vi "MeasLeakRate02.vi"() -> ()   [LabVIEW 2011]
panel:
  out "leak rate (Torr/min)":string
  out "S20":dbl
  out "S11":dbl
  out "S10":dbl
  out "S01":dbl
  out "S00":dbl
  out "A11":dbl[](array[numeric])
  out "P":dbl
  in  "first":bool=TRUE
  out "A20":dbl[](array[numeric])
  out "A10":dbl[](array[numeric])
  out "A01":dbl[](array[numeric])
  out "A00":dbl[](array[numeric])
  in  "interval (s)":dbl=0.5
  in  "stop":bool
  out "P(Torr)":string
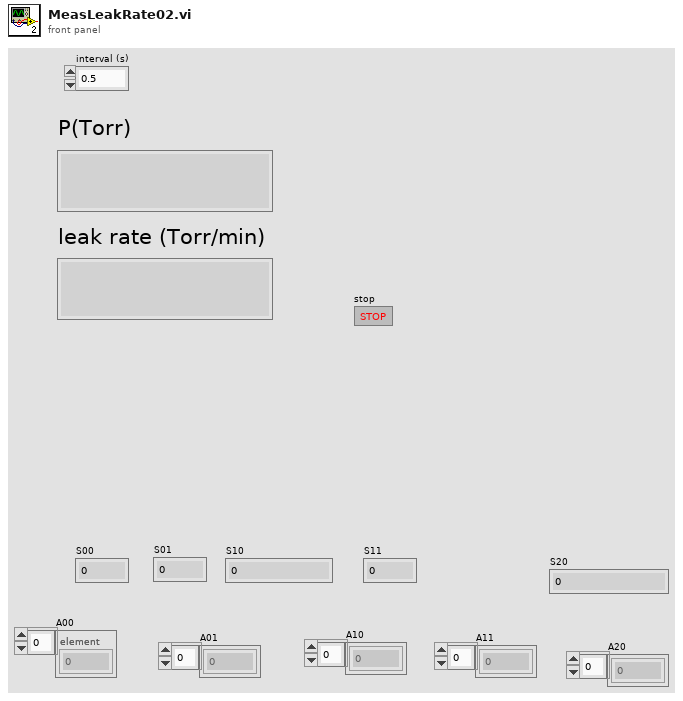
[diagram p1: front panel]
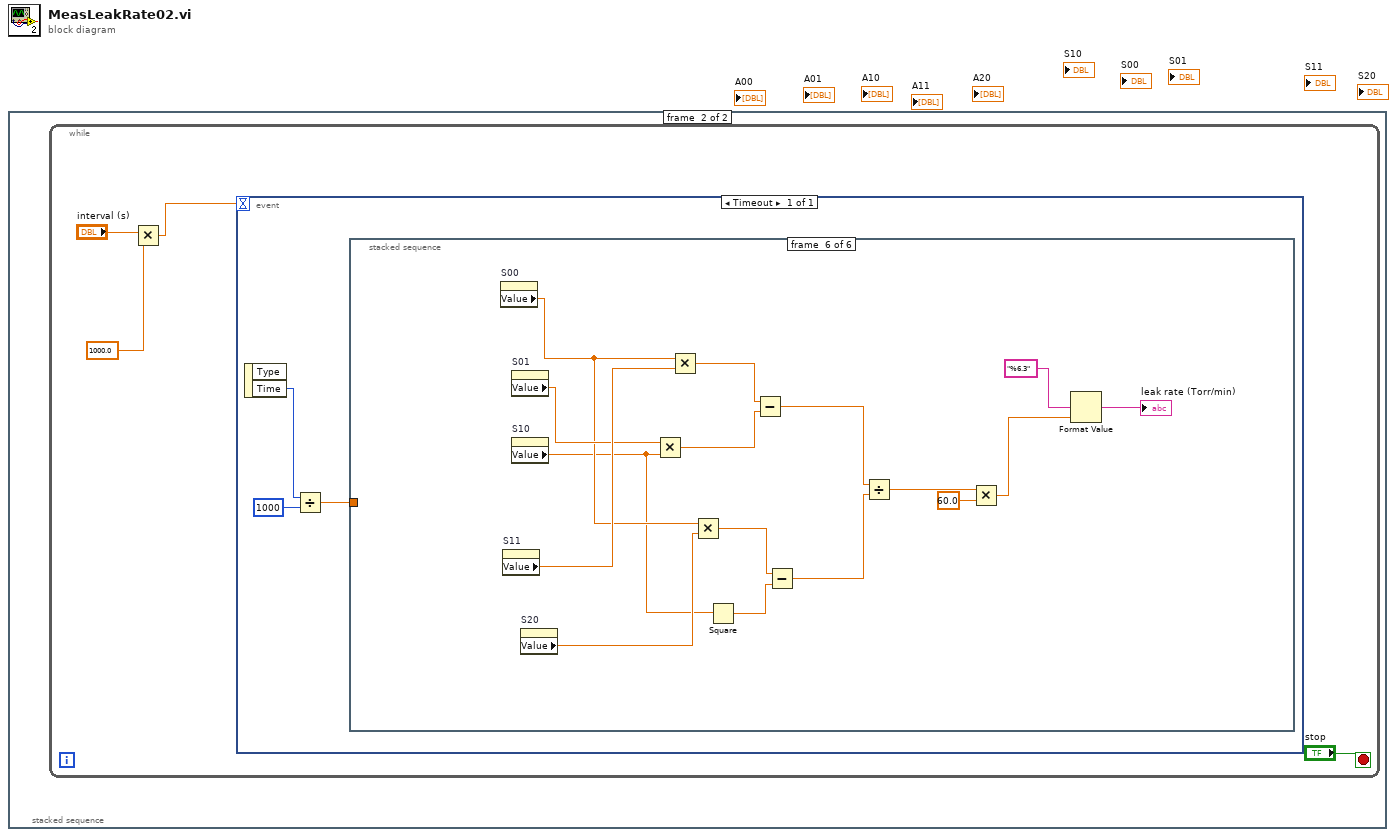
[diagram p0: block diagram]
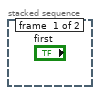
[diagram p2: hidden frame]
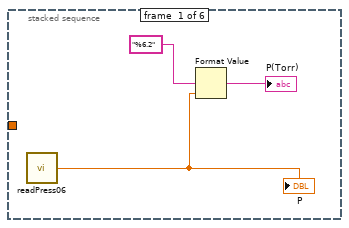
[diagram p3: hidden frame]
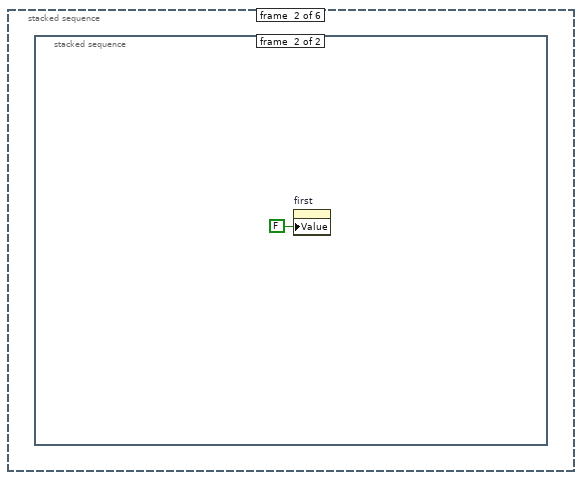
[diagram p4: hidden frame]
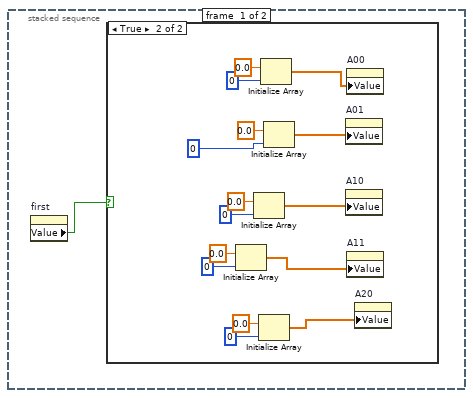
[diagram p5: hidden frame]
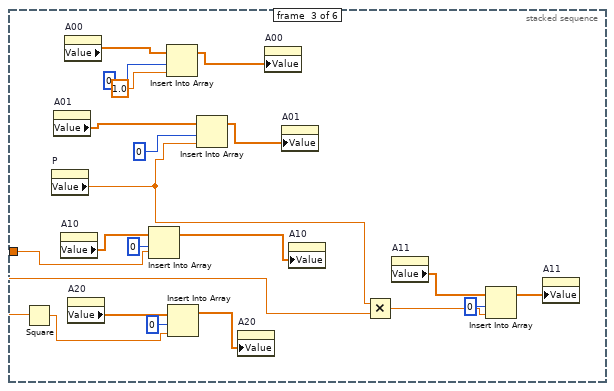
[diagram p7: hidden frame]
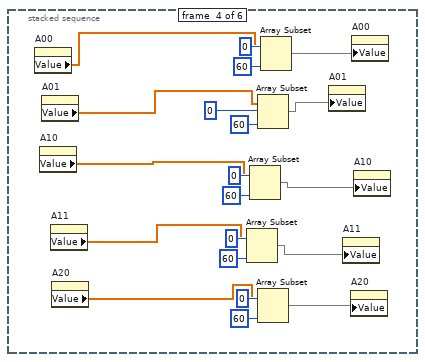
[diagram p8: hidden frame]
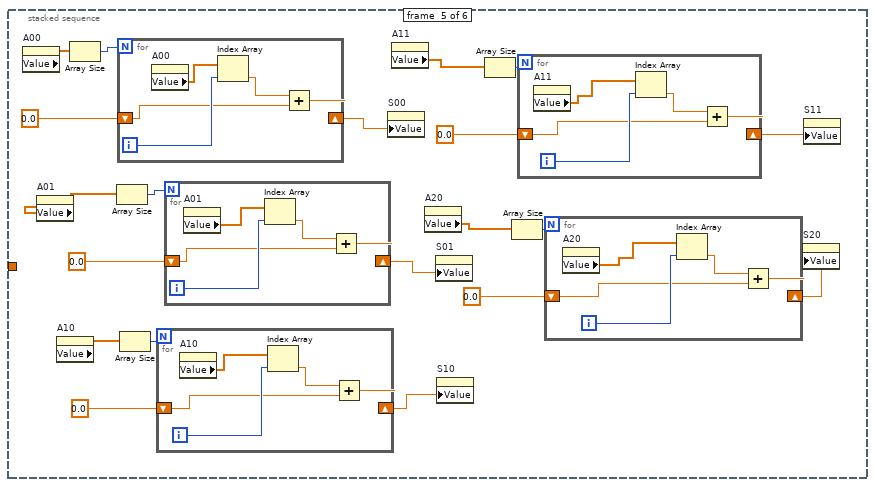
[diagram p9: hidden frame]
diagram:
  n1 = stacked-sequence {
    frame #0 {
    }
    frame #1 {
      n2 = while {
        stop <- "stop" stop-if-true
        n3 = Multiply(x="interval (s)", y=1000.0) -> (x*y=w2:dbl)
        n4 = event shown="[0] Timeout" {
          selector: _ -> [_]
          dyn-events: _ -> [_]
          timeout: w2 -> [_]
          event Timeout {
            n5 = event-data() -> ("Time"=w7:u32)  [unwired: 1 in, 1 out]
            n6 = Divide(x=w7, y=u32 1000) -> (x/y=w5:dbl)
            n7 = stacked-sequence {
              tunnel: w5 -> [_ _ w37 _ _ _]
              frame #0 {
                n8 = call "readPress06.vi"() -> ("P"=w9:dbl)
                "P" <- w9
                n9 = Format Value(format string="%6.2", value (0)=w9) -> (output string=→"P(Torr)":string)  [unwired: 1 in]
              }
              frame #1 {
                n10 = stacked-sequence {
                  frame #0 {
                    n11 = property on="first" class="Bool (strict)"() -> ("Value"=w11:bool)  [unwired: 2 in, 2 out]
                    n12 = case shown="True" w11 {
                      frame False {
                      }
                      frame True {
                        n13 = Initialize Array(0.0 ("element"), 0 ("dimension size")) -> (w14:dbl[])
                        n14 = Initialize Array(0.0 ("element"), 0 ("dimension size")) -> (w15:dbl[])
                        n15 = Initialize Array(0.0 ("element"), 0 ("dimension size")) -> (w13:dbl[])
                        n16 = Initialize Array(0.0 ("element"), 0 ("dimension size")) -> (w12:dbl[])
                        n17 = Initialize Array(0.0 ("element"), 0 ("dimension size")) -> (w16:dbl[])
                        n18 = property on="A01" class="Arr (strict)"("Value"=w16) -> ()  [unwired: 2 in, 2 out]
                        n19 = property on="A10" class="Arr (strict)"("Value"=w15) -> ()  [unwired: 2 in, 2 out]
                        n20 = property on="A00" class="Arr (strict)"("Value"=w12) -> ()  [unwired: 2 in, 2 out]
                        n21 = property on="A11" class="Arr (strict)"("Value"=w14) -> ()  [unwired: 2 in, 2 out]
                        n22 = property on="A20" class="Arr (strict)"("Value"=w13) -> ()  [unwired: 2 in, 2 out]
                      }
                    }
                  }
                  frame #1 {
                    n23 = property on="first" class="Bool (strict)"("Value"=FALSE ("first")) -> ()  [unwired: 2 in, 2 out]
                  }
                }
              }
              frame #2 {
                n24 = Square(x=w37) -> (x^2=w38:dbl)
                n25 = property on="P" class="DigNum (strict)"() -> ("Value"=w36:dbl)  [unwired: 2 in, 2 out]
                n26 = property on="A01" class="Arr (strict)"() -> ("Value"=w43:dbl[])  [unwired: 2 in, 2 out]
                n27 = property on="A10" class="Arr (strict)"() -> ("Value"=w42:dbl[])  [unwired: 2 in, 2 out]
                n28 = property on="A00" class="Arr (strict)"() -> ("Value"=w45:dbl[])  [unwired: 2 in, 2 out]
                n29 = property on="A20" class="Arr (strict)"() -> ("Value"=w40:dbl[])  [unwired: 2 in, 2 out]
                n30 = Insert Into Array(array=w42, index=0, new element=w37) -> (w30:dbl[])
                n31 = Insert Into Array(array=w45, index=0, new element=1.0 ("new element/subarray")) -> (w32:dbl[])
                n32 = Insert Into Array(array=w40, index=0, new element=w38) -> (w31:dbl[])
                n33 = Insert Into Array(array=w43, index=0, new element=w36) -> (w28:dbl[])
                n34 = property on="A20" class="Arr (strict)"("Value"=w31) -> ()  [unwired: 2 in, 2 out]
                n35 = property on="A00" class="Arr (strict)"("Value"=w32) -> ()  [unwired: 2 in, 2 out]
                n36 = property on="A01" class="Arr (strict)"("Value"=w28) -> ()  [unwired: 2 in, 2 out]
                n37 = property on="A10" class="Arr (strict)"("Value"=w30) -> ()  [unwired: 2 in, 2 out]
                n38 = Multiply(x=w36, y=w37) -> (x*y=w34:dbl)
                n39 = property on="A11" class="Arr (strict)"() -> ("Value"=w35:dbl[])  [unwired: 2 in, 2 out]
                n40 = Insert Into Array(array=w35, index=0, new element=w34) -> (w29:dbl[])
                n41 = property on="A11" class="Arr (strict)"("Value"=w29) -> ()  [unwired: 2 in, 2 out]
              }
              frame #3 {
                n42 = property on="A00" class="Arr (strict)"() -> ("Value"=w62:dbl[])  [unwired: 2 in, 2 out]
                n43 = property on="A10" class="Arr (strict)"() -> ("Value"=w53:dbl[])  [unwired: 2 in, 2 out]
                n44 = property on="A01" class="Arr (strict)"() -> ("Value"=w54:dbl[])  [unwired: 2 in, 2 out]
                n45 = property on="A11" class="Arr (strict)"() -> ("Value"=w52:dbl[])  [unwired: 2 in, 2 out]
                n46 = property on="A20" class="Arr (strict)"() -> ("Value"=w65:dbl[])  [unwired: 2 in, 2 out]
                n47 = Array Subset(array=w52, index=0, length=60) -> (w49:dbl[])
                n48 = Array Subset(array=w53, index=0, length=60) -> (w50:dbl[])
                n49 = Array Subset(array=w54, index=0, length=60) -> (w51:dbl[])
                n50 = Array Subset(array=w65, index=0, length=60) -> (w48:dbl[])
                n51 = Array Subset(array=w62, index=0, length=60) -> (w61:dbl[])
                n52 = property on="A01" class="Arr (strict)"("Value"=w51) -> ()  [unwired: 2 in, 2 out]
                n53 = property on="A11" class="Arr (strict)"("Value"=w49) -> ()  [unwired: 2 in, 2 out]
                n54 = property on="A20" class="Arr (strict)"("Value"=w48) -> ()  [unwired: 2 in, 2 out]
                n55 = property on="A00" class="Arr (strict)"("Value"=w61) -> ()  [unwired: 2 in, 2 out]
                n56 = property on="A10" class="Arr (strict)"("Value"=w50) -> ()  [unwired: 2 in, 2 out]
              }
              frame #4 {
                n57 = property on="A00" class="Arr (strict)"() -> ("Value"=w86:dbl[])  [unwired: 2 in, 2 out]
                n58 = property on="A01" class="Arr (strict)"() -> ("Value"=w82:dbl[])  [unwired: 2 in, 2 out]
                n59 = property on="A10" class="Arr (strict)"() -> ("Value"=w79:dbl[])  [unwired: 2 in, 2 out]
                n60 = Array Size(array=w86) -> (size(s)=w87:i32)
                n61 = Array Size(array=w82) -> (size(s)=w84:i32)
                n62 = for {
                  N: w87 -> [_]
                  shift-right: [w108] -> w72
                  shift-left: 0.0 -> [w109]
                  i -> [w111]
                  n63 = property on="A00" class="Arr (strict)"() -> ("Value"=w112:dbl[])  [unwired: 2 in, 2 out]
                  n64 = Index Array(array=w112, index=w111) -> (element=w110:dbl)
                  n65 = Add(x=w110, y=w109) -> (x+y=w108:dbl)
                }
                n66 = Array Size(array=w79) -> (size(s)=w81:i32)
                n67 = for {
                  N: w81 -> [_]
                  shift-right: [w99] -> w71
                  shift-left: 0.0 -> [w100]
                  i -> [w102]
                  n68 = property on="A10" class="Arr (strict)"() -> ("Value"=w98:dbl[])  [unwired: 2 in, 2 out]
                  n69 = Index Array(array=w98, index=w102) -> (element=w101:dbl)
                  n70 = Add(x=w101, y=w100) -> (x+y=w99:dbl)
                }
                n71 = for {
                  N: w84 -> [_]
                  shift-right: [w104] -> w70
                  shift-left: 0.0 -> [w105]
                  i -> [w107]
                  n72 = property on="A01" class="Arr (strict)"() -> ("Value"=w103:dbl[])  [unwired: 2 in, 2 out]
                  n73 = Index Array(array=w103, index=w107) -> (element=w106:dbl)
                  n74 = Add(x=w106, y=w105) -> (x+y=w104:dbl)
                }
                n75 = property on="S00" class="DigNum (strict)"("Value"=w72) -> ()  [unwired: 2 in, 2 out]
                n76 = property on="A11" class="Arr (strict)"() -> ("Value"=w76:dbl[])  [unwired: 2 in, 2 out]
                n77 = property on="A20" class="Arr (strict)"() -> ("Value"=w73:dbl[])  [unwired: 2 in, 2 out]
                n78 = property on="S01" class="DigNum (strict)"("Value"=w70) -> ()  [unwired: 2 in, 2 out]
                n79 = property on="S10" class="DigNum (strict)"("Value"=w71) -> ()  [unwired: 2 in, 2 out]
                n80 = Array Size(array=w76) -> (size(s)=w78:i32)
                n81 = Array Size(array=w73) -> (size(s)=w75:i32)
                n82 = for {
                  N: w78 -> [_]
                  shift-right: [w94] -> w69
                  shift-left: 0.0 -> [w95]
                  i -> [w97]
                  n83 = property on="A11" class="Arr (strict)"() -> ("Value"=w93:dbl[])  [unwired: 2 in, 2 out]
                  n84 = Index Array(array=w93, index=w97) -> (element=w96:dbl)
                  n85 = Add(x=w96, y=w95) -> (x+y=w94:dbl)
                }
                n86 = for {
                  N: w75 -> [_]
                  shift-right: [w89] -> w68
                  shift-left: 0.0 -> [w90]
                  i -> [w92]
                  n87 = property on="A20" class="Arr (strict)"() -> ("Value"=w88:dbl[])  [unwired: 2 in, 2 out]
                  n88 = Index Array(array=w88, index=w92) -> (element=w91:dbl)
                  n89 = Add(x=w91, y=w90) -> (x+y=w89:dbl)
                }
                n90 = property on="S20" class="DigNum (strict)"("Value"=w68) -> ()  [unwired: 2 in, 2 out]
                n91 = property on="S11" class="DigNum (strict)"("Value"=w69) -> ()  [unwired: 2 in, 2 out]
              }
              frame #5 {
                n92 = property on="S00" class="DigNum (strict)"() -> ("Value"=w124:dbl)  [unwired: 2 in, 2 out]
                n93 = property on="S11" class="DigNum (strict)"() -> ("Value"=w128:dbl)  [unwired: 2 in, 2 out]
                n94 = property on="S01" class="DigNum (strict)"() -> ("Value"=w127:dbl)  [unwired: 2 in, 2 out]
                n95 = property on="S10" class="DigNum (strict)"() -> ("Value"=w122:dbl)  [unwired: 2 in, 2 out]
                n96 = property on="S20" class="DigNum (strict)"() -> ("Value"=w123:dbl)  [unwired: 2 in, 2 out]
                n97 = Multiply(x=w127, y=w122) -> (x*y=w125:dbl)
                n98 = Multiply(x=w124, y=w128) -> (x*y=w126:dbl)
                n99 = Multiply(x=w124, y=w123) -> (x*y=w121:dbl)
                n100 = Square(x=w122) -> (x^2=w120:dbl)
                n101 = Subtract(x=w126, y=w125) -> (x-y=w119:dbl)
                n102 = Subtract(x=w121, y=w120) -> (x-y=w118:dbl)
                n103 = Divide(x=w119, y=w118) -> (x/y=w117:dbl)
                n104 = Multiply(x=w117, y=60.0) -> (x*y=w113:dbl)
                n105 = Format Value(format string="%6.3", value (0)=w113) -> (output string=→"leak rate (Torr/min)":string)  [unwired: 1 in]
              }
            }
          }
        }
      }
    }
  }
